vi "Pre-Build Action (Pharlap x86).vi"(6 "Top Level/Always Included VIs":path[](array[path]), 7 "Main Destination Path":path, 9 "Target Name":string, 10 "Build Specification Name":string, 11 "Project Path":path) -> (0 "error out":errorcluster)   [LabVIEW 2017]
uses:
  Development Tools/Build Automation/Build Automation.lvlib
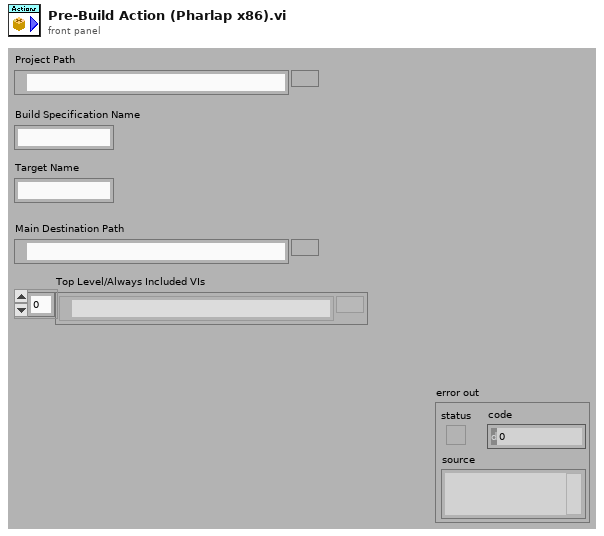
[diagram p1: front panel]
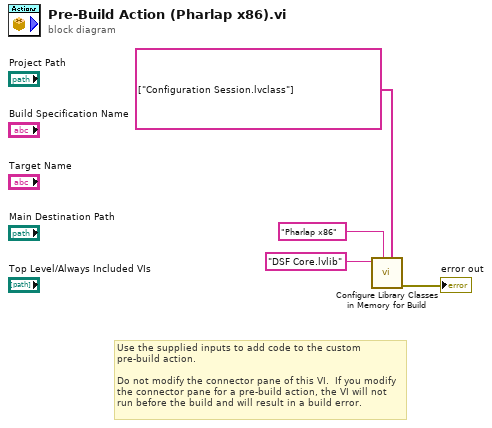
[diagram p0: block diagram]
diagram:
  # "Use the supplied inputs to add code to the custom pre-build action.\n\nDo not modify the connector pane of this VI.  If you modify the connector pane for a pre-build action, the VI will not run before the build and will result in a build error."
  n1 = call "Configure Library Classes in Memory for Build.vi"("skip inline classes"=string[] ["Configuration Session.lvclass"], "target name (My Computer)"="Pharlap x86", "library name"="DSF Core.lvlib") -> ("error out"=→"error out":errorcluster)  [unwired: 8 in]
